vi "MB Write Single Hold Registers.vi"(8 "error in (no error)":errorcluster, 9 "Write Hold Register":u16, 10 "Control Variable":string, 11 "Devices":T1) -> (0 "error out":errorcluster, 3 "Devices out":T1)   [LabVIEW 2021]
uses:
  <vilib>/NI/Modbus Library/API/Master/Modbus Master.lvclass
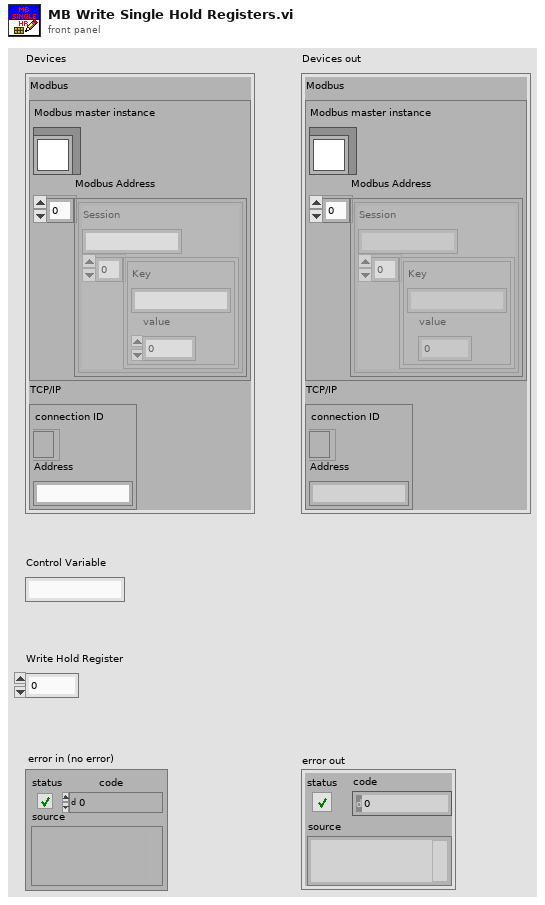
[diagram p1: front panel]
types:
  T1 = cluster{"Modbus":cluster{"Modbus master instance":refnum<class "Modbus Master.lvclass">, "Modbus Address":cluster{"Session":string, cluster{"Key":string, "value":u32}[]}[]}, "TCP/IP":cluster{"connection ID":refnum<k5>, "Address":string}}
  T2 = cluster{"Session":string, cluster{"Key":string, "value":u32}[]}[]
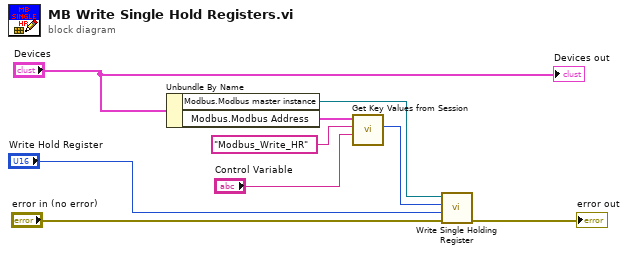
[diagram p0: block diagram]
diagram:
  n1 = Unbundle By Name("Devices") -> ("Modbus.Modbus master instance"=w9:refnum<class "Modbus Master.lvclass">, "Modbus.Modbus Address"=w4:T2)
  n2 = call "Get Key Values from Session.vi"("Key"="Control Variable", "Session"="Modbus_Write_HR", "Ini File"=w4) -> ("Search Key Value"=w1:u32)  [unwired: 6 in, 2 out]
  n3 = call-dynamic "Write Single Holding Register.vi"("error in"="error in (no error)", "register to write"="Write Hold Register", "address"=w1, "Modbus master in"=w9) -> ("error out"=→"error out":errorcluster)  [unwired: 6 in, 1 out]
  "Devices out" <- "Devices"
